vi "Set configuration chain.vi"(8 "error in (no error)":errorcluster, 9 "class names":string[](array[string]), 10 "configuration":variant[](array[variant]), 11 "ExampleClassDScaffold in":refnum<class "ExampleClassDScaffold.lvclass">) -> (0 "error out":errorcluster, 3 "ExampleClassDScaffold out":refnum<class "ExampleClassDScaffold.lvclass">)   [LabVIEW 2012, in "ExampleClassDScaffold.lvclass"]
uses:
  ExampleClassDScaffold.lvclass
  <vilib>/Distrio/Murmex/Murmex/Murmex.lvclass
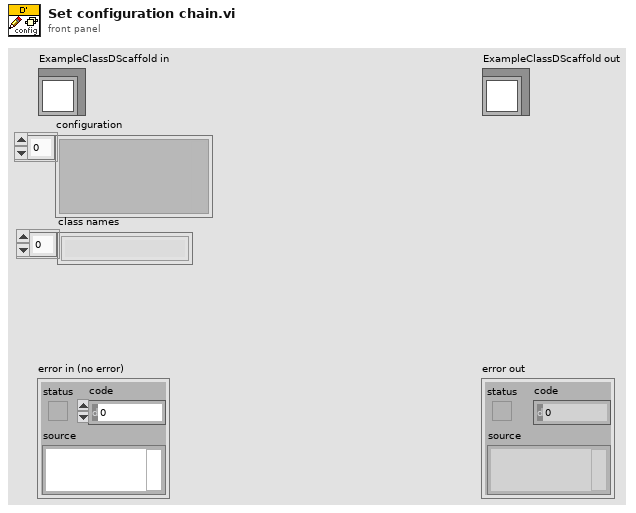
[diagram p1: front panel]
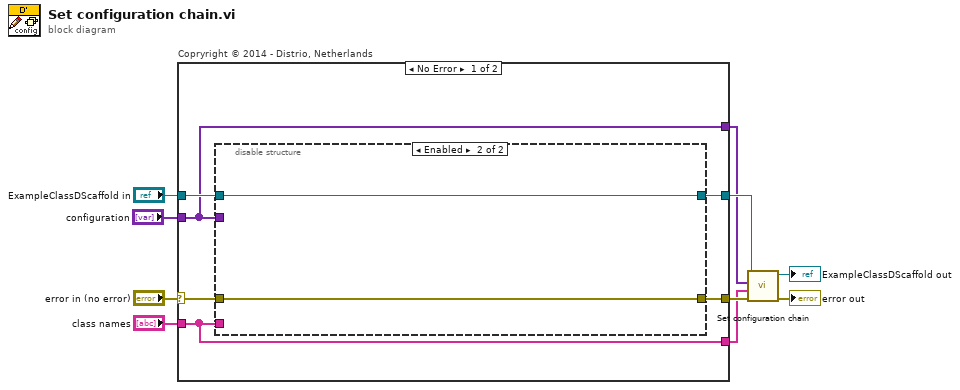
[diagram p0: block diagram]
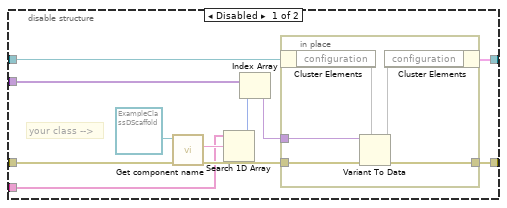
[diagram p2: hidden frame]
diagram:
  n1 = case "Copryright © 2014 - Distrio, Netherlands" shown="No Error" "error in (no error)" {
    selector: "error in (no error)" -> [w16 w36]
    tunnel: [w13 w36] -> w4
    tunnel: [w14 w35] -> w5
    tunnel: "ExampleClassDScaffold in" -> [w15 w35]
    tunnel: "class names" -> [w12 _]
    tunnel: "configuration" -> [w11 _]
    tunnel: [w12 _] -> w2
    tunnel: [w11 _] -> w1
    frame No Error {
      n2 = disable-structure shown="Enabled" {
        disable-tunnel: w16 -> [w27 w33]
        disable-tunnel: w11 -> [w25 _]
        disable-tunnel: w15 -> [w21 w34]
        disable-tunnel: [w20 w34] -> w14
        disable-tunnel: [w19 w33] -> w13
        disable-tunnel: w12 -> [w18 _]
        frame Disabled {
          # "your class -->"
          n3 = call <vilib>:"Get component name.vi"("error in (no error)"=w27, "Murmex in"=refnum<class "ExampleClassDScaffold.lvclass"> refnum ("ExampleClassDScaffold in")) -> ("error out"=w22:errorcluster, "component name"=w26:string)  [unwired: 7 in, 1 out]
          n4 = Search 1D Array(1D array=w18, element=w26) -> (index of element=w24:i32)  [unwired: 1 in]
          n5 = Index Array(array=w25, index=w24) -> (element=w23:variant)
          n6 = in-place {
            in-place-border: w23 -> [w32]
            in-place-border: w22 -> [w30]
            in-place-border: [w28] -> w19
            n7 = in-place-cluster #1(w21) -> ("configuration"=w31)
            n8 = Variant To Data(error in=w30, type=w31, Variant=w32) -> (data=w29, error out=w28:errorcluster)
            n9 = in-place-cluster #1("configuration"=w29) -> (w20:cluster{})
          }
        }
        frame Enabled {
        }
      }
    }
    frame Error {
    }
  }
  n10 = call-parent "Set configuration chain.vi"("error in (no error)"=w4, "class names"=w2, "configuration"=w1, "Murmex in"=w5) -> ("error out"=→"error out":errorcluster, "Murmex out"=→"ExampleClassDScaffold out":refnum<class "ExampleClassDScaffold.lvclass">)  [unwired: 6 in]
